vi "LookAhead.vi"(8 "error in (no error)":errorcluster, 10 "Index":i32, 11 "JSON String":string) -> (0 "error out":errorcluster, 1 "TOKEN":T1, 2 "Index Passthrough":i32, 3 "JSON String Passthrough":string)   [LabVIEW 2017, in "JSON Support for LabVIEW.lvlib"]
uses:
  JSON Support for LabVIEW.lvlib
  Token Type.ctl
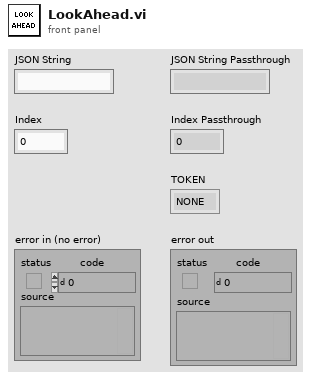
[diagram p1: front panel]
types:
  T1 = typedef "JSON Support for LabVIEW.lvlib/Token Type.ctl" = enum16{"NONE", "CURLY_OPEN", "CURLY_CLOSE", "SQUARED_OPEN", "SQUARED_CLOSE", "COLON", "COMMA", "STRING", "NUMBER", "TRUE", "FALSE", "NULL"}
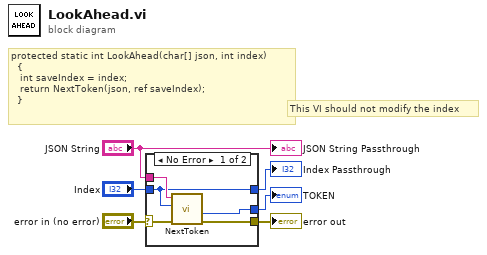
[diagram p0: block diagram]
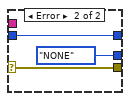
[diagram p2: hidden frame]
diagram:
  # "This VI should not modify the index"
  # "protected static int LookAhead(char[] json, int index)\n\t\t{\n\t\t\tint saveIndex = index;\n\t\t\treturn NextToken(json, ref saveIndex);\n\t\t}"
  n1 = case shown="No Error" "error in (no error)" {
    selector: "error in (no error)" -> [w9 w14]
    tunnel: [w8 w14] -> w5
    tunnel: "JSON String" -> [w11 _]
    tunnel: [w10 w13] -> w3
    tunnel: "Index" -> [w10 w13]
    tunnel: [w7 Token_Type."NONE" ("TOKEN")] -> w1
    frame No Error {
      n2 = call "NextToken.vi"("error in (no error)"=w9, "Index In"=w10, "JSON String"=w11) -> ("error out"=w8:errorcluster, "TOKEN"=w7:T1)  [unwired: 5 in, 2 out]
    }
    frame Error {
    }
  }
  "error out" <- w5
  "Index Passthrough" <- w3
  "TOKEN" <- w1
  "JSON String Passthrough" <- "JSON String"
